vi "runPushing.vi"(4 "Service? in":bool, 5 "Distance":dbl, 6 "Fault?":bool, 7 "Time":dbl, 8 "error in (no error)":errorcluster, 9 "Actuators in":T1, 10 "State in":T2, 11 "RunType in":refnum<class "RunType.lvclass">) -> (0 "error out":errorcluster, 1 "Actuators out":T1, 2 "State out":T2, 3 "RunType out":refnum<class "RunType.lvclass">)   [LabVIEW 2018, in "ControlLibrary.lvlib" / "RunType.lvclass"]
uses:
  RunType.lvclass
  TypeDef_ControlState.ctl
  TypeDef_DigitalOuts.ctl
  RunType.lvclass/RunType.ctl
  TypeDef_RunParameters.ctl
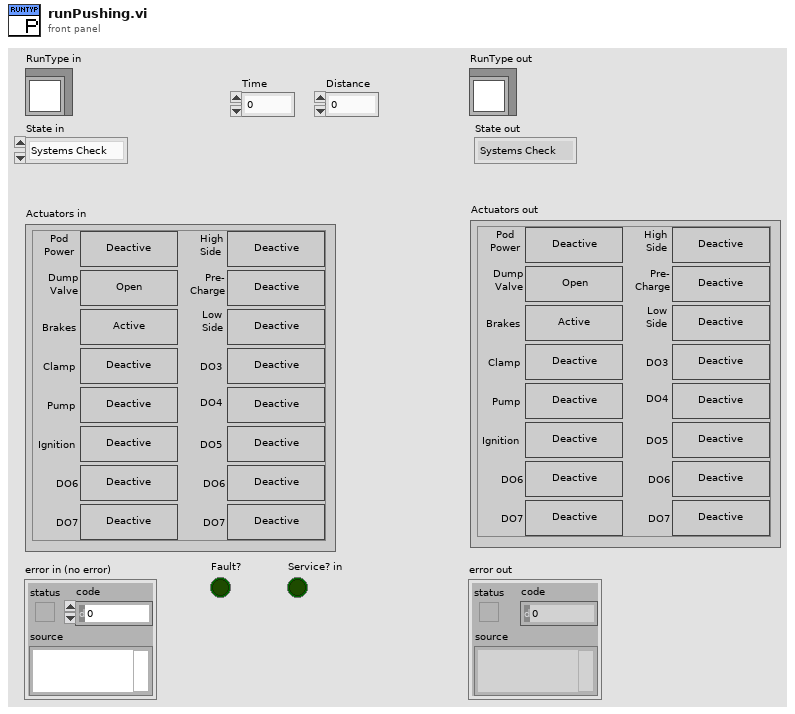
[diagram p1: front panel]
types:
  T1 = typedef "TypeDef_DigitalOuts.ctl" = cluster{"Pod Power":bool, "Dump Valve":bool, "Brakes":bool, "Clamp":bool, "Pump":bool, "Ignition":bool, "DO6":bool, "DO7":bool, "HighSide":bool, "Precharge":bool, "LowSide":bool, "DO3":bool, "DO4":bool, "DO5":bool, "DO62":bool, "DO72":bool}
  T2 = typedef "TypeDef_ControlState.ctl" = enum16{"Systems Check", "Idle", "Ready", "Pushing", "Coast", "Braking", "Fault", "Shutdown", "Service", "Precharge", "Blank"}
  T3 = typedef "TypeDef_RunParameters.ctl" = cluster{"Distance Threshold (ft)":dbl, "Time Threshold (s)":dbl, "Target (I16)":i16}
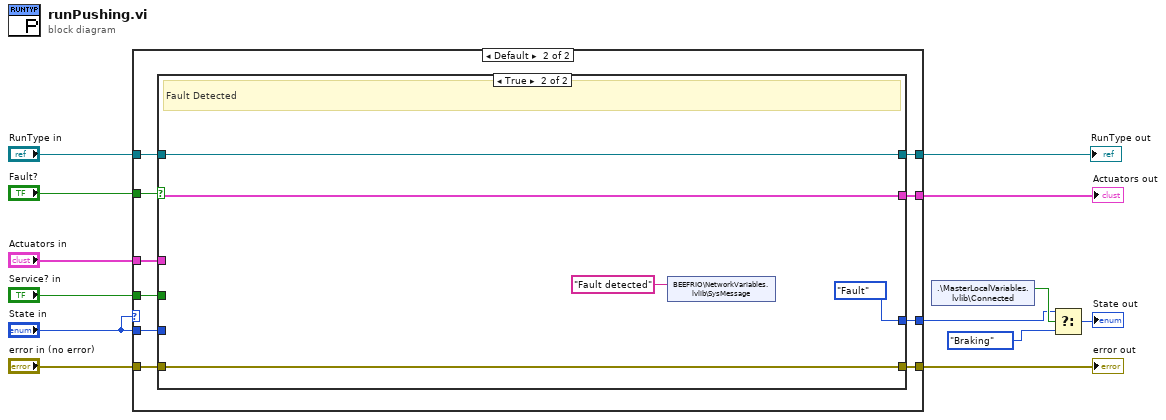
[diagram p0: block diagram]
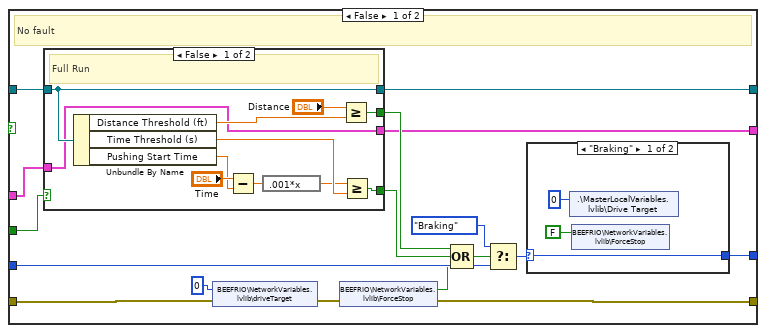
[diagram p3: hidden frame]
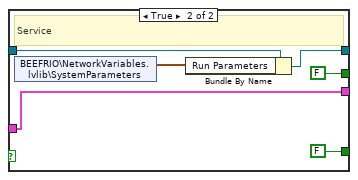
[diagram p4: hidden frame]
diagram:
  n1 = case shown="Default" "State in" {
    tunnel: "error in (no error)" -> [w14 w27]
    tunnel: [w14 w26] -> w12
    tunnel: "State in" -> [w15 w25]
    tunnel: [w15 w24] -> w3
    tunnel: "Fault?" -> [_ w23]
    tunnel: "RunType in" -> [w17 w22]
    tunnel: "Service? in" -> [_ w21]
    tunnel: [w17 w20] -> w8
    tunnel: "Actuators in" -> [w16 w19]
    tunnel: [w16 w18] -> w6
    frame "Braking" {
    }
    frame Default {
      n2 = case shown="True" w23 {
        tunnel: w27 -> [w29 w70]
        tunnel: [w44 w70] -> w26
        tunnel: w25 -> [w43 _]
        tunnel: [w42 TypeDef_ControlState."Fault" ("State in")] -> w24
        tunnel: w22 -> [w39 w68]
        tunnel: w21 -> [w34 _]
        tunnel: [w33 w68] -> w20
        tunnel: w19 -> [w32 w67]
        tunnel: [w31 w67] -> w18
        frame False {
          # "No fault"
          n3 = case shown="False" w34 {
            tunnel: w39 -> [w50 w59]
            tunnel: [w52 FALSE] -> w38
            tunnel: [w51 FALSE] -> w37
            tunnel: [w50 w58] -> w33
            tunnel: w32 -> [w45 w56]
            tunnel: [w45 w56] -> w31
            frame False {
              # "Full Run"
              n4 = Unbundle By Name(w50) -> ("Distance Threshold (ft)"=w54:dbl, "Time Threshold (s)"=w53:dbl, "Pushing Start Time"=w48:dbl)
              n5 = Subtract(x="Time", y=w48) -> (x-y=w47:dbl)
              n6 = expression code=".001*x"(w47) -> (w46:dbl)
              n7 = Greater Or Equal?(x="Distance", y=w54) -> (x >= y?=w52:bool)
              n8 = Greater Or Equal?(x=w46, y=w53) -> (x >= y?=w51:bool)
            }
            frame True {
              # "Service"
              n9 = shared-variable "BEEFRIO\\NetworkVariables.lvlib\\SystemParameters"() -> (w57:T3)  [unwired: 1 in, 1 out]
              n10 = Bundle By Name(cluster=w59, "Run Parameters"=w57) -> (w58:refnum<class "RunType.lvclass">)
            }
          }
          n11 = shared-variable "BEEFRIO\\NetworkVariables.lvlib\\driveTarget"(i16 0 ("driveTarget"), error in=w29) -> (error out=w28:errorcluster)
          n12 = shared-variable "BEEFRIO\\NetworkVariables.lvlib\\ForceStop"(error in=w28) -> (w36:bool, error out=w44:errorcluster)
          n13 = Compound Arithmetic op=OR(w38, w37, w36) -> (w35:bool)
          n14 = Select(t=TypeDef_ControlState."Braking", s=w35, f=w43) -> (s? t:f=w40:T2)
          n15 = case shown="\"Braking\"" w40 {
            selector: w40 -> [w64 w65]
            tunnel: [w64 w65] -> w42
            frame "Braking" {
              n16 = shared-variable ".\\MasterLocalVariables.lvlib\\Drive Target"(i16 0 ("driveTarget")) -> ()  [unwired: 1 in, 1 out]
              n17 = shared-variable "BEEFRIO\\NetworkVariables.lvlib\\ForceStop"(FALSE ("ForceStop")) -> ()  [unwired: 1 in, 1 out]
            }
            frame Default {
            }
          }
        }
        frame True {
          # "Fault Detected"
          n18 = shared-variable "BEEFRIO\\NetworkVariables.lvlib\\SysMessage"("Fault detected" ("SysMessage")) -> ()  [unwired: 1 in, 1 out]
        }
      }
    }
  }
  "error out" <- w12
  "RunType out" <- w8
  "Actuators out" <- w6
  n19 = shared-variable ".\\MasterLocalVariables.lvlib\\Connected"() -> (w4:bool)  [unwired: 1 in, 1 out]
  n20 = Select(t=w3, s=w4, f=TypeDef_ControlState."Braking") -> (s? t:f=→"State out":T2)
